vi "DAQParametersRef.vi"(2 "DAQ Device IN":T1={"DAQ Fs (S/s)"=10000.0, "task"="", "error"={"status"=FALSE, "code"=0, "source"=""}, "Min Value"=-10.0, "Max Value"=10.0}, 3 "DAQ Controls":refnum<vi>) -> (0 "DAQ Device OUT":T1, 1 "En Funcionamiento?":bool)   [LabVIEW 2010]
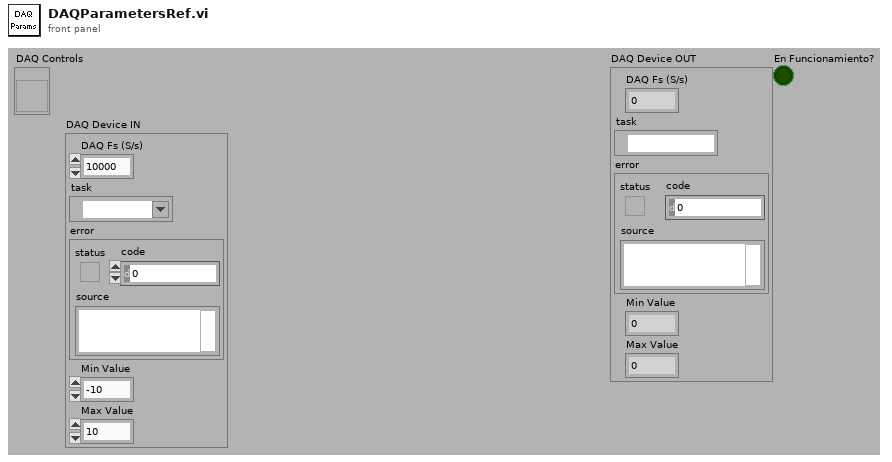
[diagram p1: front panel]
types:
  T1 = cluster{"DAQ Fs (S/s)":dbl, "task":refnum<k21>, "error":errorcluster, "Min Value":dbl, "Max Value":dbl}
  T2 = cluster{"Minimum Value":dbl, "Maximum Value":dbl, "Physical Channel":tag, "DAQ Fs (S/s)":dbl}
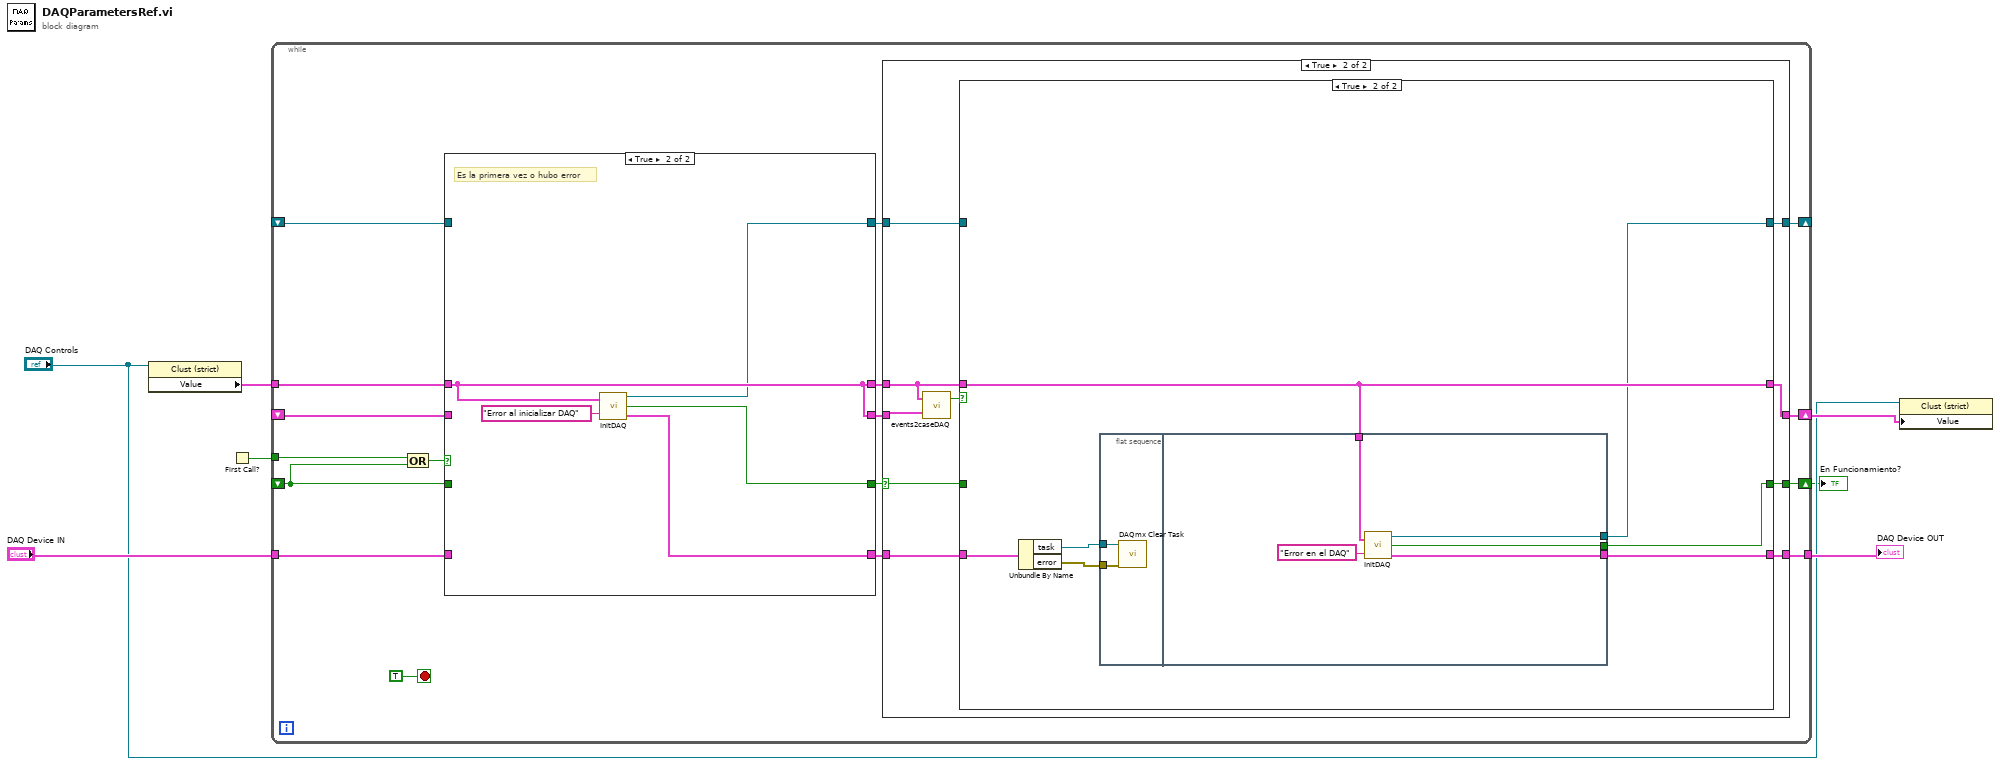
[diagram p0: block diagram]
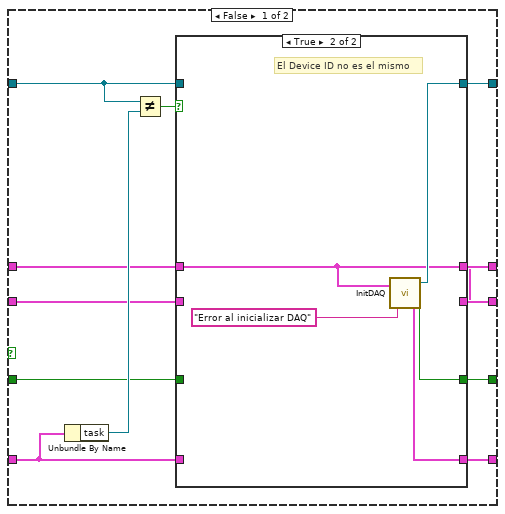
[diagram p4: hidden frame]
diagram:
  n1 = property class="Clust (strict)"(reference="DAQ Controls") -> ("Value"=w6:T2)  [unwired: 1 in, 2 out]
  n2 = First Call?() -> (First Call?: T/F=w7:bool)
  n3 = while {
    tunnel: w6 -> [w20]
    shift-right: [w23] -> w3
    shift-left: _ -> [w19]
    tunnel: "DAQ Device IN" -> [w11]
    tunnel: [w22] -> w4
    tunnel: w7 -> [w12]
    shift-right: [w13] -> _
    shift-left: _ -> [w16]
    shift-right: [w8] -> w1
    shift-left: _ -> [w10]
    stop <- TRUE stop-if-true
    n4 = Compound Arithmetic op=OR(w12, w10) -> (w15:bool)
    n5 = case shown="True" w15 {
      tunnel: [w61 w80] -> w14
      tunnel: [w63 w82] -> w21
      tunnel: w20 -> [w64 w82]
      tunnel: w19 -> [w59 _]
      tunnel: [w62 w82] -> w18
      tunnel: [w68 w81] -> w17
      tunnel: w11 -> [w67 _]
      tunnel: w16 -> [w57 _]
      tunnel: [w60 w83] -> w9
      tunnel: w10 -> [w58 _]
      frame False {
        n6 = Unbundle By Name(w67) -> ("task"=w66:refnum<k21>)
        n7 = Not Equal?(x=w57, y=w66) -> (x != y?=w65:bool)
        n8 = case shown="True" w65 {
          tunnel: [w73 w76] -> w68
          tunnel: w67 -> [w73 _]
          tunnel: w64 -> [w72 w75]
          tunnel: [w72 w75] -> w63
          tunnel: [w71 w75] -> w62
          tunnel: [w69 w78] -> w61
          tunnel: [w70 w77] -> w60
          tunnel: w59 -> [w71 _]
          tunnel: w58 -> [w70 _]
          tunnel: w57 -> [w69 _]
          frame False {
            # "Sigue siendo todo igual"
          }
          frame True {
            # "El Device ID no es el mismo"
            n9 = call "InitDAQ.vi"("message"="Error al inicializar DAQ", "DAQ Parameters"=w75) -> ("DAQ Device OUT"=w76:T1, "Inicializo DAQ?"=w77:bool, "task OUT"=w78:refnum<k21>)
          }
        }
      }
      frame True {
        # "Es la primera vez o hubo error"
        n10 = call "InitDAQ.vi"("message"="Error al inicializar DAQ", "DAQ Parameters"=w82) -> ("DAQ Device OUT"=w81:T1, "Inicializo DAQ?"=w83:bool, "task OUT"=w80:refnum<k21>)
      }
    }
    n11 = case shown="True" w9 {
      selector: w9 -> [w25 w30]
      tunnel: [w28 w37] -> w23
      tunnel: [w27 w36] -> w22
      tunnel: w14 -> [w26 w35]
      tunnel: w21 -> [w28 w29]
      tunnel: w18 -> [_ w32]
      tunnel: w17 -> [w27 w34]
      tunnel: [w26 w33] -> w13
      tunnel: [w25 w31] -> w8
      frame False {
      }
      frame True {
        n12 = call "events2caseDAQ.vi"("DAQ Controls Old"=w32, "DAQ Controls New"=w29) -> ("DAQ Cambio?"=w38:bool)  [unwired: 1 out]
        n13 = case shown="True" w38 {
          tunnel: [w42 w46] -> w37
          tunnel: w29 -> [w42 w46]
          tunnel: w34 -> [w41 w49]
          tunnel: [w41 w43] -> w36
          tunnel: w35 -> [w40 _]
          tunnel: [w40 w45] -> w33
          tunnel: [w39 w44] -> w31
          tunnel: w30 -> [w39 _]
          frame False {
          }
          frame True {
            n14 = Unbundle By Name(w49) -> ("task"=w47:refnum<k21>, "error"=w48:errorcluster)
            n15 = flat-sequence {
              tunnel: w47 -> [w51]
              tunnel: w48 -> [w50]
              tunnel: w46 -> [w55]
              tunnel: [w54] -> w45
              tunnel: [w53] -> w44
              tunnel: [w52] -> w43
              frame #0 {
                n16 = call <vilib>:"DAQmx Clear Task.vi"("task in"=w51, "error in"=w50) -> ()  [unwired: 13 in, 1 out]
              }
              frame #1 {
                n17 = call "InitDAQ.vi"("message"="Error en el DAQ", "DAQ Parameters"=w55) -> ("DAQ Device OUT"=w52:T1, "Inicializo DAQ?"=w53:bool, "task OUT"=w54:refnum<k21>)
              }
            }
          }
        }
      }
    }
  }
  "DAQ Device OUT" <- w4
  "En Funcionamiento?" <- w1
  n18 = property class="Clust (strict)"(reference="DAQ Controls", "Value"=w3) -> ()  [unwired: 1 in, 2 out]
